vi "Create Coverage Report - Uncovered Diagrams - Appear as Uncovered Branches.vi"() -> ()   [LabVIEW 2017, in "Cobertura.Tests.lvlib"]
uses:
  Cobertura.Tests.lvlib
  Cobertura/Coverage/Coverage.lvclass/Coverage.ctl
  Cobertura/Package/Package.lvclass/Package.ctl
  Cobertura/Class/Class.lvclass/Class.ctl
  Cobertura/Method/Method.lvclass/Method.ctl
  Cobertura/Line/Line.lvclass/Line.ctl
  Cobertura/Coverage/Read Packages.vi
  Cobertura/Package/Read Classes.vi
  Cobertura/Class/Read Methods.vi
  Cobertura/Method/Read Lines.vi
  Cobertura/Line/Read Branch.vi
  Cobertura/Line/Read Condition Coverage.vi
  Fake Project Inspector/Fake Project Inspector.lvclass
  C:/Users/Pascal/Projects/Home/lvunit/Cobertura/Project Inspector Base/Project Inspector Base.lvclass
  Fake Code Coverage/Fake Code Coverage.lvclass
  C:/Users/Pascal/Projects/Home/lvunit/Code Coverage/Code Coverage.lvclass
  Fake Code Inspector/Fake Code Inspector.lvclass
  C:/Users/Pascal/Projects/Home/lvunit/Cobertura/Code Inspector Base/Code Inspector Base.lvclass
  Cobertura/Package/Package.lvclass
  Cobertura/Class/Class.lvclass
  Cobertura/Method/Method.lvclass
  Cobertura/Line/Line.lvclass
  Cobertura/Cobertura.lvlib
  <vilib>/PNR/Transparent Assertions/Transparent Assertions/Transparent Assertions.lvlib
  Cobertura/Coverage/Coverage.lvclass
panel:
  out "error out":errorcluster
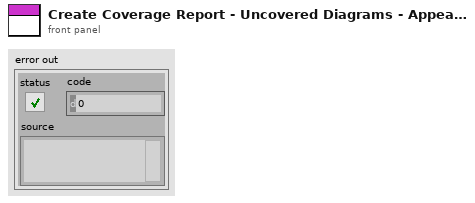
[diagram p1: front panel]
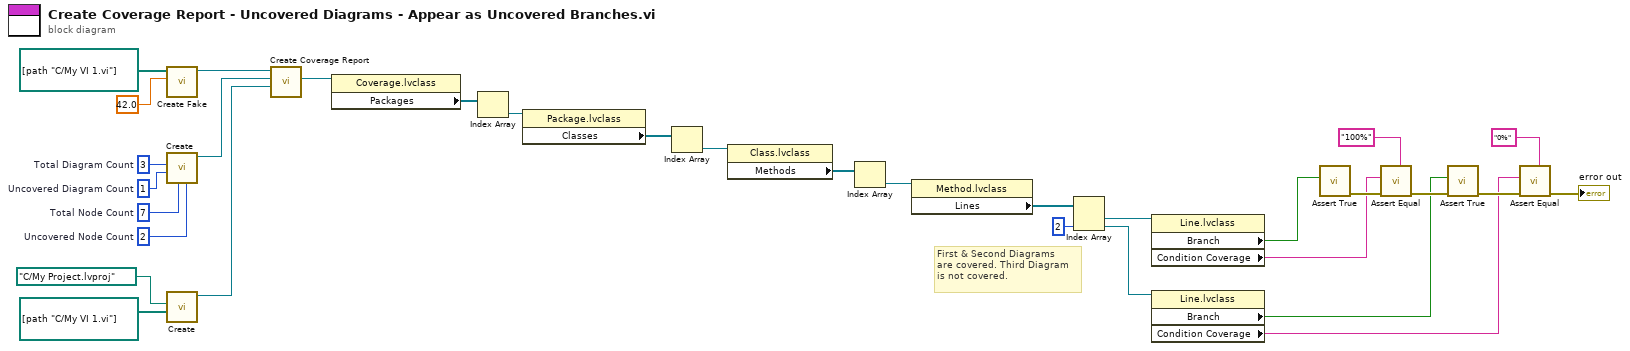
[diagram p0: block diagram]
diagram:
  w15 = 2  # Uncovered Node Count
  w16 = 7  # Total Node Count
  w17 = 1  # Uncovered Diagram Count
  w18 = 3  # Total Diagram Count
  # "First & Second Diagrams\nare covered. Third Diagram\nis not covered."
  n1 = call "Create Fake.vi"("Coverage Percentage"=42.0, "All VIs Measured"=path[] [path "C:/My VI 1.vi"] ("Item Paths")) -> ("Fake Code Coverage"=w22:refnum<class "Fake Code Coverage.lvclass">)  [unwired: 8 in, 1 out]
  n2 = call "Create.vi"("Uncovered Node Count"=w15, "Total Node Count"=w16, "Uncovered Diagram Count"=w17, "Total Diagram Count"=w18) -> ("Fake Code Inspector"=w19:refnum<class "Fake Code Inspector.lvclass">)  [unwired: 6 in, 1 out]
  n3 = call "Create.vi"("Item Paths"=path[] [path "C:/My VI 1.vi"], "Path"=path "C:/My Project.lvproj") -> ("Fake Project Inspector"=w30:refnum<class "Fake Project Inspector.lvclass">)  [unwired: 8 in, 1 out]
  n4 = call "Create Coverage Report.vi"("Project Inspector"=w30, "Code Inspector"=w19, "CodeCoverage in"=w22) -> ("Coverage"=w32:refnum<class "Coverage.lvclass">)  [unwired: 7 in, 1 out]
  n5 = property class="Coverage.lvclass"(reference=w32) -> ("Packages"=w31:refnum<class "Package.lvclass">[])  [unwired: 1 in, 2 out]
  n6 = Index Array(array=w31) -> (element=w28:refnum<class "Package.lvclass">)  [unwired: 1 in]
  n7 = property class="Package.lvclass"(reference=w28) -> ("Classes"=w27:refnum<class "Class.lvclass">[])  [unwired: 1 in, 2 out]
  n8 = Index Array(array=w27) -> (element=w25:refnum<class "Class.lvclass">)  [unwired: 1 in]
  n9 = property class="Class.lvclass"(reference=w25) -> ("Methods"=w24:refnum<class "Method.lvclass">[])  [unwired: 1 in, 2 out]
  n10 = Index Array(array=w24) -> (element=w23:refnum<class "Method.lvclass">)  [unwired: 1 in]
  n11 = property class="Method.lvclass"(reference=w23) -> ("Lines"=w14:refnum<class "Line.lvclass">[])  [unwired: 1 in, 2 out]
  n12 = Index Array(array=w14, index #2=2 ("index")) -> (element #1=w13:refnum<class "Line.lvclass">, element #2=w12:refnum<class "Line.lvclass">)  [unwired: 1 in]
  n13 = property class="Line.lvclass"(reference=w13) -> ("Branch"=w11:bool, "Condition Coverage"=w9:string)  [unwired: 1 in, 2 out]
  n14 = property class="Line.lvclass"(reference=w12) -> ("Branch"=w7:bool, "Condition Coverage"=w5:string)  [unwired: 1 in, 2 out]
  n15 = call <vilib>:"Assert True.vi"("Condition"=w11) -> ("error out"=w10:errorcluster)  [unwired: 10 in]
  n16 = call <vilib>:"Assert Equal.vi"("Expected"="100%" ("Condition Coverage"), "error in (no error)"=w10, "Actual"=w9) -> ("error out"=w8:errorcluster)  [unwired: 8 in]
  n17 = call <vilib>:"Assert True.vi"("error in (no error)"=w8, "Condition"=w7) -> ("error out"=w6:errorcluster)  [unwired: 9 in]
  n18 = call <vilib>:"Assert Equal.vi"("Expected"="0%" ("Condition Coverage"), "error in (no error)"=w6, "Actual"=w5) -> ("error out"=→"error out":errorcluster)  [unwired: 8 in]
